vi "Initialize1287.vi"(0 "VISA Name In":refnum<visa-resource-name>="Solartron1287", 1 "Operation Mode":bool=TRUE, 2 "Overload Action":string(combo)="OL0", 3 "DC Bias":string="PC0" caption="PCF (Amps)\nPVF (Volts)", 4 "Internal Resistor":string(combo)="RR6", 5 "Error In (No Error)":errorcluster, 6 "Bandwidth":string(combo)="2", 7 "Bias Rejection ON?":bool, 8 "Voltage Gain":string(combo)="VX0", 9 "Bias Reject Mode":bool, 10 "Current Gain":string(combo)="IX0", 11 "Fixed Voltage Rejection":string="VR0", 12 "Perturbation Waveform Gain":string(combo)="PI1", 13 "Fixed Current Rejection":string="IR0") -> (14 "VISA Name Out":refnum<visa-resource-name>, 15 "Pol Gain Correction":dbl, 17 "I Gain Correction":dbl, 18 "V Gain Correction":dbl, 19 "Error Out":errorcluster)   [LabVIEW 2018]
panel:
  # "Inputs"
  # "Outputs"
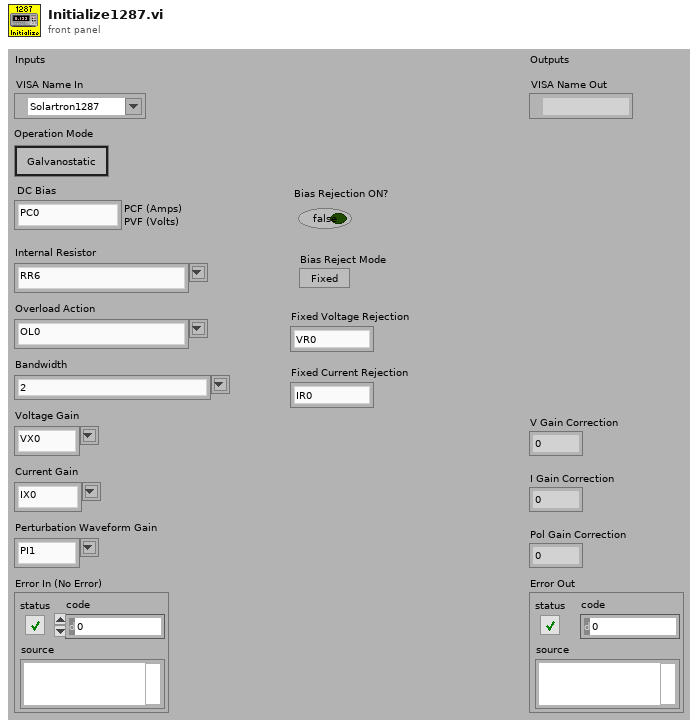
[diagram p1: front panel]
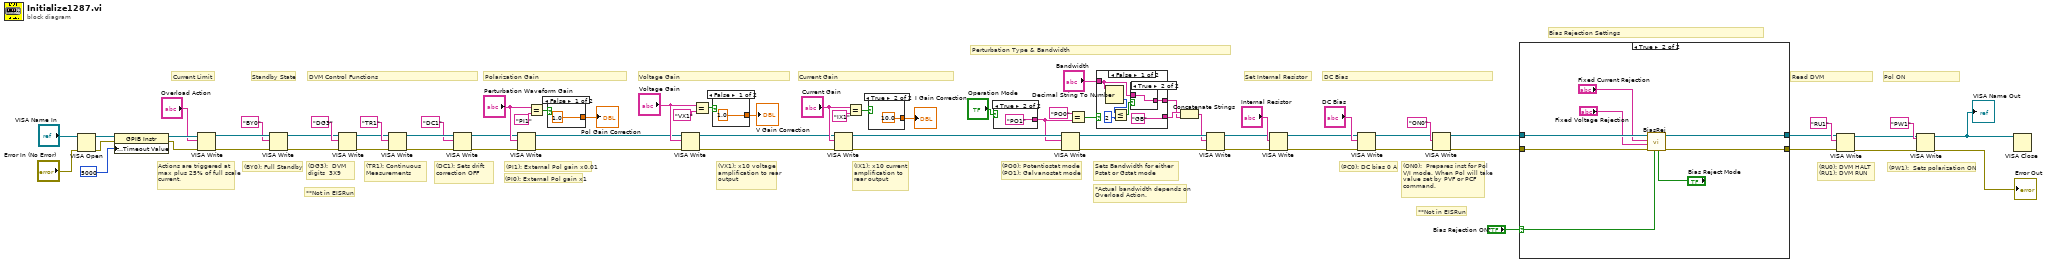
[diagram p0: block diagram]
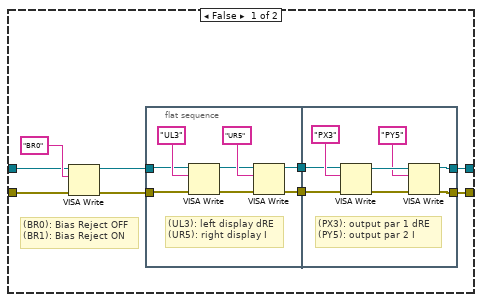
[diagram p2: hidden frame]
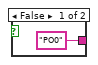
[diagram p3: hidden frame]
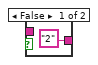
[diagram p4: hidden frame]
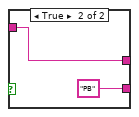
[diagram p5: hidden frame]
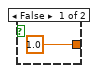
[diagram p6: hidden frame]
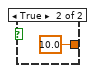
[diagram p7: hidden frame]
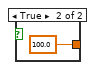
[diagram p8: hidden frame]
diagram:
  # "Bias Rejection Settings"
  # "Pol ON"
  # "Read DVM"
  # "(RU0): DVM HALT\n(RU1): DVM RUN"
  # "**Not in EISRun"
  # "(DG3):  DVM digits  3X9"
  # "Perturbation Type & Bandwidth"
  # "(PC0): DC bias 0 A"
  # "*Actual bandwidth depends on Overload Action."
  # "Sets Bandwidth for either Pstat or Gstat mode"
  # "(PO0): Potentiostat mode\n(PO1): Galvanostat mode"
  # "Current Gain"
  # "Voltage Gain"
  # "**Not in EISRun"
  # "(PW1):  Sets polarization ON"
  # "(ON0):  Prepares inst for Pol V/I mode. When Pol will take value set by PVF or PCF command."
  # "DC Bias"
  # "(IX1): x10 current amplification to rear output"
  # "(VX1): x10 voltage amplification to rear  output"
  # "Set Internal Resistor"
  # "Polarization Gain"
  # "(PI0): External Pol gain x1"
  # "(PI1): External Pol gain x0.01"
  # "(DC1): Sets drift correction OFF"
  # "DVM Control Functions"
  # "(TR1): Continuous Measurements"
  # "(BY0): Full Standby"
  # "Standby State"
  # "Actions are triggered at max plus 25% of full scale current."
  # "Current Limit"
  n1 = VISA Open(error in (no error)="Error In (No Error)", VISA resource name="VISA Name In") -> (VISA resource name=w68:refnum<visa-resource-name>, error out=w67:errorcluster)  [unwired: 3 in]
  n2 = property class="GPIB Instr"(reference=w68, error in=w67, "General Settings:Timeout Value"=u32 5000) -> (reference out=w66:refnum<visa-resource-name>, error out=w65:errorcluster)
  n3 = VISA Write(VISA resource name=w66, write buffer="Overload Action", error in (no error)=w65) -> (VISA resource name out=w63:refnum<visa-resource-name>, error out=w62:errorcluster)  [unwired: 1 out]
  n4 = VISA Write(VISA resource name=w63, write buffer="BY0", error in (no error)=w62) -> (VISA resource name out=w22:refnum<visa-resource-name>, error out=w20:errorcluster)  [unwired: 1 out]
  n5 = VISA Write(VISA resource name=w22, write buffer="DG3", error in (no error)=w20) -> (VISA resource name out=w21:refnum<visa-resource-name>, error out=w19:errorcluster)  [unwired: 1 out]
  n6 = VISA Write(VISA resource name=w21, write buffer="TR1", error in (no error)=w19) -> (VISA resource name out=w59:refnum<visa-resource-name>, error out=w58:errorcluster)  [unwired: 1 out]
  n7 = VISA Write(VISA resource name=w59, write buffer="DC1", error in (no error)=w58) -> (VISA resource name out=w52:refnum<visa-resource-name>, error out=w51:errorcluster)  [unwired: 1 out]
  n8 = VISA Write(VISA resource name=w52, write buffer="Perturbation Waveform Gain", error in (no error)=w51) -> (VISA resource name out=w29:refnum<visa-resource-name>, error out=w28:errorcluster)  [unwired: 1 out]
  n9 = Equal?(x="Perturbation Waveform Gain", y="PI1") -> (x = y?=w54:bool)
  n10 = case shown="False" w54 {
    tunnel: [1.0 100.0] -> w50
    frame False {
    }
    frame True {
    }
  }
  "Pol Gain Correction" <- w50
  n11 = VISA Write(VISA resource name=w29, write buffer="Voltage Gain", error in (no error)=w28) -> (VISA resource name out=w37:refnum<visa-resource-name>, error out=w36:errorcluster)  [unwired: 1 out]
  n12 = Equal?(x="Voltage Gain", y="VX1") -> (x = y?=w47:bool)
  n13 = case shown="False" w47 {
    tunnel: [1.0 10.0] -> w46
    frame False {
    }
    frame True {
    }
  }
  "V Gain Correction" <- w46
  n14 = VISA Write(VISA resource name=w37, write buffer="Current Gain", error in (no error)=w36) -> (VISA resource name out=w27:refnum<visa-resource-name>, error out=w26:errorcluster)  [unwired: 1 out]
  n15 = Equal?(x="Current Gain", y="IX1") -> (x = y?=w44:bool)
  n16 = case shown="True" w44 {
    tunnel: [1.0 10.0] -> w43
    frame False {
    }
    frame True {
    }
  }
  "I Gain Correction" <- w43
  n17 = case shown="True" "Operation Mode" {
    tunnel: ["PO0" "PO1"] -> w8
    frame False {
    }
    frame True {
    }
  }
  n18 = VISA Write(VISA resource name=w27, write buffer=w8, error in (no error)=w26) -> (VISA resource name out=w34:refnum<visa-resource-name>, error out=w35:errorcluster)  [unwired: 1 out]
  n19 = Equal?(x="PO0", y=w8) -> (x = y?=w31:bool)
  n20 = case shown="False" w31 {
    tunnel: "Bandwidth" -> [w81 w88]
    tunnel: ["GB" "PB"] -> w12
    tunnel: [w79 w88] -> w11
    frame False {
      n21 = Decimal String To Number(string=w81) -> (number=w82:i32)  [unwired: 2 in, 1 out]
      n22 = Less Or Equal?(x=w82, y=2) -> (x <= y?=w83:bool)
      n23 = case shown="True" w83 {
        tunnel: ["2" ("GPIB\nAddress") w86] -> w79
        tunnel: w81 -> [_ w86]
        frame False {
        }
        frame True {
        }
      }
    }
    frame True {
    }
  }
  n24 = Concatenate Strings(w12, w11) -> (w33:string)
  n25 = VISA Write(VISA resource name=w34, write buffer=w33, error in (no error)=w35) -> (VISA resource name out=w25:refnum<visa-resource-name>, error out=w24:errorcluster)  [unwired: 1 out]
  n26 = VISA Write(VISA resource name=w25, write buffer="Internal Resistor", error in (no error)=w24) -> (VISA resource name out=w7:refnum<visa-resource-name>, error out=w6:errorcluster)  [unwired: 1 out]
  n27 = VISA Write(VISA resource name=w7, write buffer="DC Bias", error in (no error)=w6) -> (VISA resource name out=w18:refnum<visa-resource-name>, error out=w17:errorcluster)  [unwired: 1 out]
  n28 = VISA Write(VISA resource name=w18, write buffer="ON0", error in (no error)=w17) -> (VISA resource name out=w5:refnum<visa-resource-name>, error out=w4:errorcluster)  [unwired: 1 out]
  n29 = case shown="True" "Bias Rejection ON?" {
    selector: "Bias Rejection ON?" -> [_ w115]
    tunnel: w5 -> [w96 w121]
    tunnel: w4 -> [w95 w120]
    tunnel: [w90 w118] -> w3
    tunnel: [w89 w119] -> w2
    frame False {
      # "(BR0): Bias Reject OFF\n(BR1): Bias Reject ON"
      n30 = VISA Write(VISA resource name=w96, write buffer="BR0" ("data"), error in (no error)=w95) -> (VISA resource name out=w94:refnum<visa-resource-name>, error out=w93:errorcluster)  [unwired: 1 out]
      n31 = flat-sequence {
        tunnel: w94 -> [w101]
        tunnel: w93 -> [w100]
        tunnel: [w99] -> w92
        tunnel: [w98] -> w91
        tunnel: w92 -> [w106]
        tunnel: w91 -> [w107]
        tunnel: [w109] -> w90
        tunnel: [w108] -> w89
        frame #0 {
          # "(UL3): left display dRE\n(UR5): right display I"
          n32 = VISA Write(VISA resource name=w101, write buffer="UL3" ("y"), error in (no error)=w100) -> (VISA resource name out=w103:refnum<visa-resource-name>, error out=w102:errorcluster)  [unwired: 1 out]
          n33 = VISA Write(VISA resource name=w103, write buffer="UR5" ("y"), error in (no error)=w102) -> (VISA resource name out=w98:refnum<visa-resource-name>, error out=w99:errorcluster)  [unwired: 1 out]
        }
        frame #1 {
          # "(PX3): output par 1 dRE\n(PY5): output par 2 I"
          n34 = VISA Write(VISA resource name=w107, write buffer="PX3" ("y"), error in (no error)=w106) -> (VISA resource name out=w112:refnum<visa-resource-name>, error out=w113:errorcluster)  [unwired: 1 out]
          n35 = VISA Write(VISA resource name=w112, write buffer="PY5" ("y"), error in (no error)=w113) -> (VISA resource name out=w109:refnum<visa-resource-name>, error out=w108:errorcluster)  [unwired: 1 out]
        }
      }
    }
    frame True {
      n36 = call "BiasRej.vi"("Bias Reject Mode"="Bias Reject Mode", "BiasRejectON?"=w115, "Error In (No Error)"=w120, "Fixed Voltage Rejection"="Fixed Voltage Rejection", "Fixed Current Rejection"="Fixed Current Rejection", "Potentiostat"=w121) -> ("Error Out"=w119:errorcluster, "VISA Name Out"=w118:refnum<visa-resource-name>)  [unwired: 4 in]
    }
  }
  n37 = VISA Write(VISA resource name=w3, write buffer="RU1", error in (no error)=w2) -> (VISA resource name out=w16:refnum<visa-resource-name>, error out=w15:errorcluster)  [unwired: 1 out]
  n38 = VISA Write(VISA resource name=w16, write buffer="PW1", error in (no error)=w15) -> (VISA resource name out=w14:refnum<visa-resource-name>, error out=→"Error Out":errorcluster)  [unwired: 1 out]
  "VISA Name Out" <- w14
  n39 = VISA Close(VISA resource name=w14) -> ()  [unwired: 1 in, 1 out]
